vi "Array Pile-up Correction [[SGL]].vi"(8 "Error In":errorcluster, 9 "Pixel well capacity":sgl, 11 "Image Pixels":sgl[][](array[numeric])) -> (0 "Error Out":errorcluster, 1 "# Replacements":i32, 3 "Corrected Image Pixels":sgl[][](array[numeric]))   [LabVIEW 2021, in "Arrays.lvlib"]
doc: "Computes the pile-up corrected values according to the following formula:\n\npucA[i] = -M*Ln(1-A[i]/M)\n\nwhere M is the <B>Pixel Well Capacity</b>, A[i] are the <B>Image Pixels</B> values and pucA[i] are the <B>Corrected Image Pixels</B>.\n\nIf <B>Replace Inf by NaN</B> is True, replaces +/-Inf returned values by NaN.\n\nAn error is returned if any of the <B>Image Pixels</B> is not positive or is larger than the <B>Pixel Well Capacity</B>."
uses:
  Arrays.lvlib
  9b0dc1ca-5c4f-4dbc-9472-a7971718c0ce.vi
  <vilib>/Utility/error.llb/Error Cluster From Error Code.vi
  <vilib>/ErrorRing/Error Ring.xnode
  Error/Error.lvlib
panel:
  # "see the AlliGator License on the block diagram (Ctrl+E or Window:Show Block Diagram)"
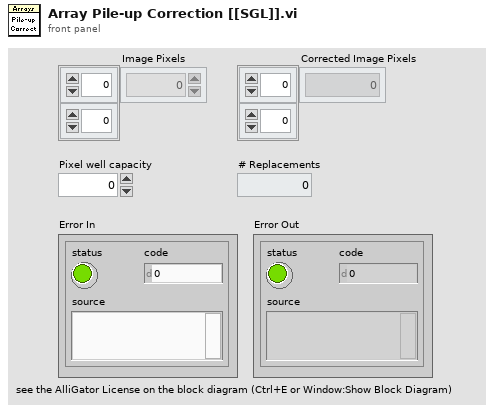
[diagram p1: front panel]
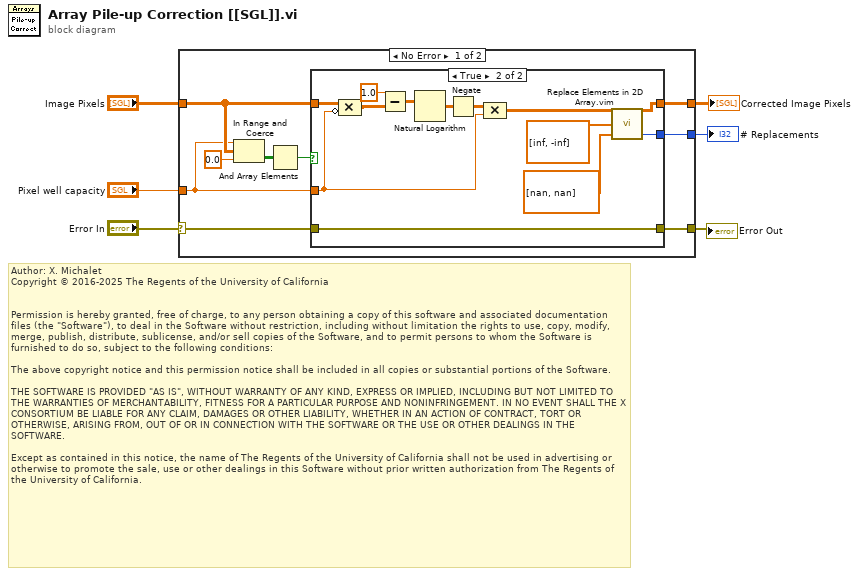
[diagram p0: block diagram]
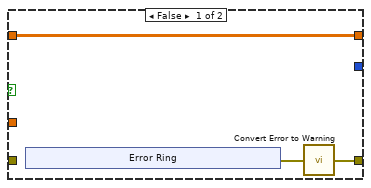
[diagram p2: hidden frame]
diagram:
  # "Author: X. Michalet\nCopyright © 2016-2025 The Regents of the University of California\n \n\nPermission is hereby granted, free of charge, to any person obtaining a copy of this software and associated documentation files (the \"Software\"), to deal in the Software without restriction, including without limitation the rights to use, copy, modify, merge, publish, distribute, sublicense, and/or sell copies of the Software, and to permit persons to whom the Software is furnished to do so, subject to the following conditions:\n\nThe above copyright notice and this permission notice shall be included in all copies or substantial portions of the Software.\n\nTHE SOFTWARE IS PROVIDED \"AS IS\", WITHOUT WARRANTY OF ANY KIND, EXPRESS OR IMPLIED, INCLUDING BUT NOT LIMITED TO THE WARRANTIES OF MERCHANTABILITY, FITNESS FOR A PARTICULAR PURPOSE AND NONINFRINGEMENT. IN NO EVENT SHALL THE X CONSORTIUM BE LIABLE FOR ANY CLAIM, DAMAGES OR OTHER LIABILITY, WHETHER IN AN ACTION OF CONTRACT, TORT OR OTHERWISE, ARISING FROM, OUT OF OR IN CONNECTION WITH THE SOFTWARE OR THE USE OR OTHER DEALINGS IN THE SOFTWARE.\n\nExcept as contained in this notice, the name of The Regents of the University of California shall not be used in advertising or otherwise to promote the sale, use or other dealings in this Software without prior written authorization from The Regents of the University of California."
  n1 = case shown="No Error" "Error In" {
    selector: "Error In" -> [w7 w36]
    tunnel: [w15 _] -> w2
    tunnel: "Pixel well capacity" -> [w11 _]
    tunnel: [w14 w37] -> w1
    tunnel: "Image Pixels" -> [w12 w37]
    tunnel: [w8 w36] -> w3
    frame No Error {
      n2 = In Range and Coerce(upper limit=w11, x=w12, lower limit=sgl 0.0) -> (In Range?=w10:bool[][])  [unwired: 1 out]
      n3 = And Array Elements(Boolean array=w10) -> (logical AND=w9:bool)
      n4 = case shown="True" w9 {
        tunnel: [_ w35] -> w15
        tunnel: [w18 w32] -> w14
        tunnel: w12 -> [w18 w26]
        tunnel: w11 -> [_ w24]
        tunnel: [w16 w25] -> w8
        tunnel: w7 -> [_ w25]
        frame False {
          n5 = xnode "Error Ring"() -> ("error out"=w17:errorcluster)
          n6 = call "Convert Error to Warning.vi"("Error In"=w17) -> ("no Error Out"=w16:errorcluster)  [unwired: 8 in]
        }
        frame True {
          n7 = Compound Arithmetic op=MULTIPLY(w26, invert w24) -> (w29:sgl[][])
          n8 = Subtract(x=sgl 1.0, y=w29) -> (x-y=w30:sgl[][])
          n9 = Natural Logarithm(1:w30) -> (0:w27:sgl[][])
          n10 = Negate(x=w27) -> (-x=w28:sgl[][])
          n11 = Compound Arithmetic op=MULTIPLY(w28, w24) -> (w31:sgl[][])
          n12 = call "Replace Elements in 2D Array.vim"("Array"=w31, "Values to Replace"=sgl[] [inf, -inf], "Replacement Values"=sgl[] [nan, nan] ("Values to Replace")) -> ("Modified Array"=w32:sgl[][], "# Replacements"=w35:i32)  [unwired: 5 in]
        }
      }
    }
    frame Error {
    }
  }
  "# Replacements" <- w2
  "Corrected Image Pixels" <- w1
  "Error Out" <- w3
